vi "S2C_Access_MenuAct.vi"(8 "Error In":errorcluster, 11 "Coords":cluster{"Row":dbl, "Column":dbl}) -> (0 "Error Out":errorcluster, 2 "MenuItems":string[](array[string]), 3 "Discard?":bool)   [LabVIEW 2015]
uses:
  S2C_Access_Globals.vi
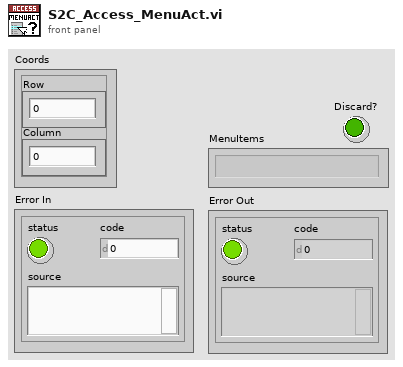
[diagram p1: front panel]
types:
  T1 = typedef "LVRowAndColumnTypeDef.ctl" = cluster{"Row":i32, "Column":i32}
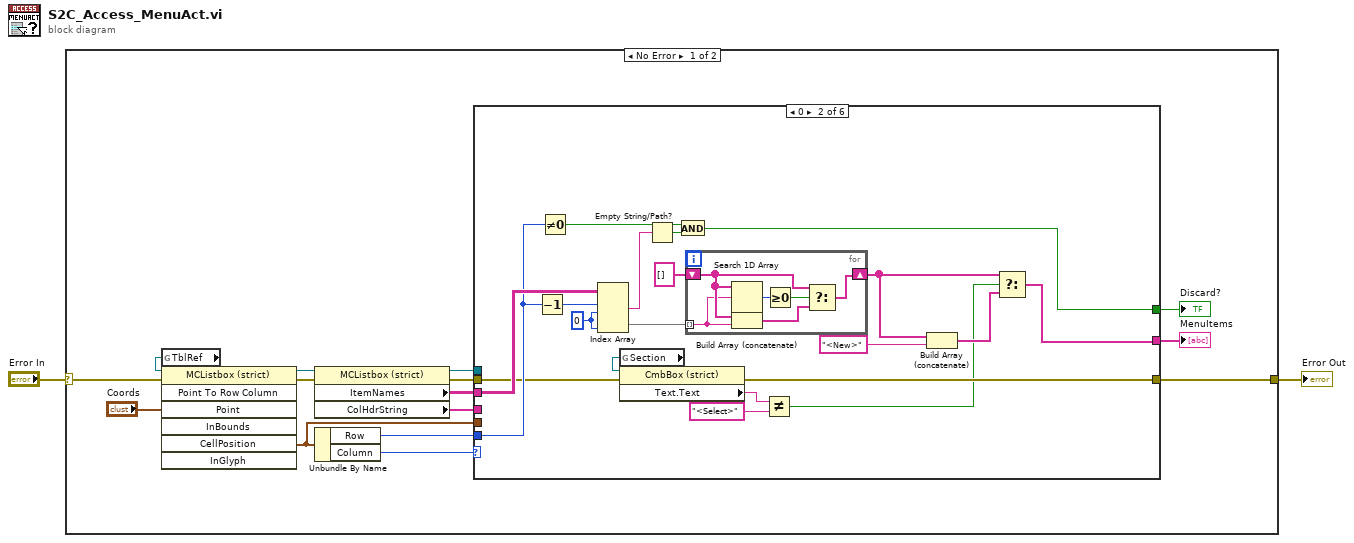
[diagram p0: block diagram]
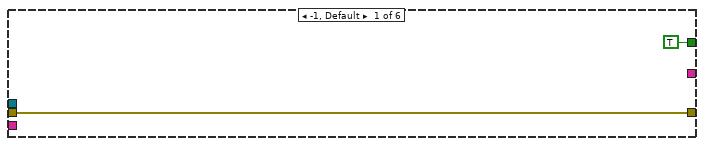
[diagram p2: hidden frame]
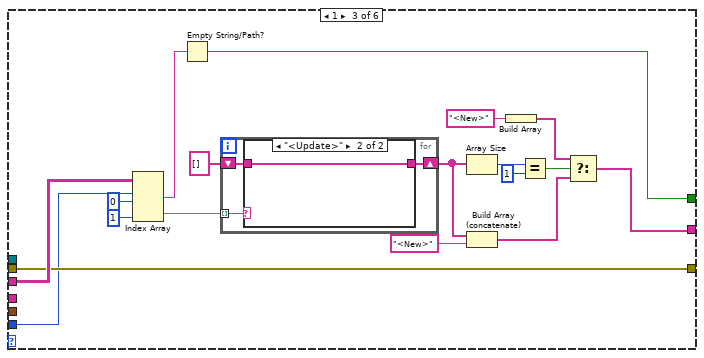
[diagram p3: hidden frame]
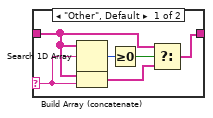
[diagram p4: hidden frame]
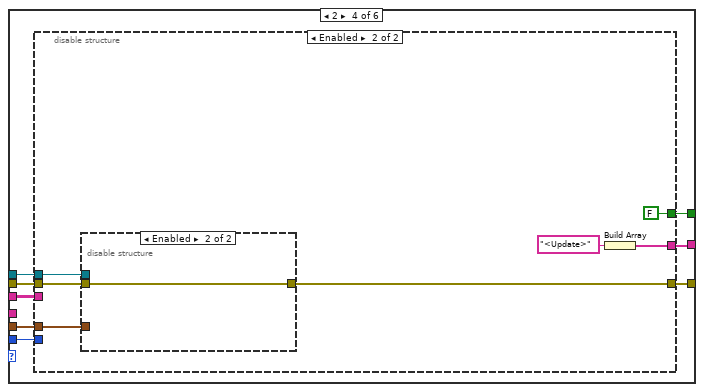
[diagram p5: hidden frame]
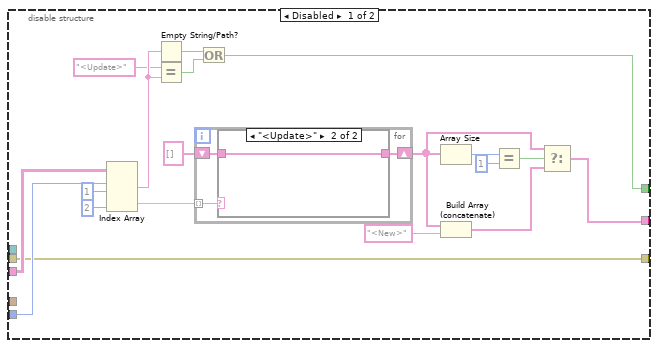
[diagram p6: hidden frame]
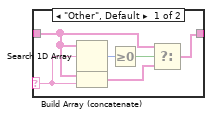
[diagram p7: hidden frame]
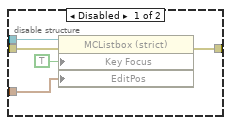
[diagram p8: hidden frame]
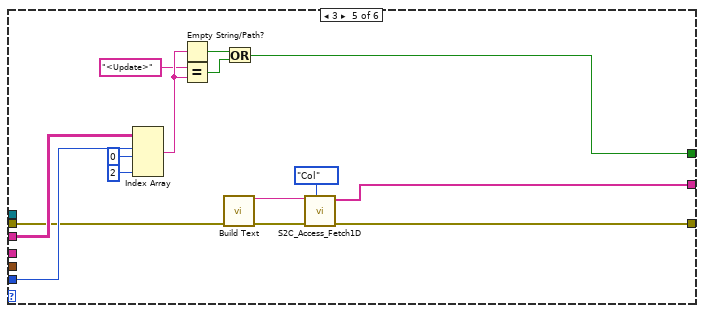
[diagram p9: hidden frame]
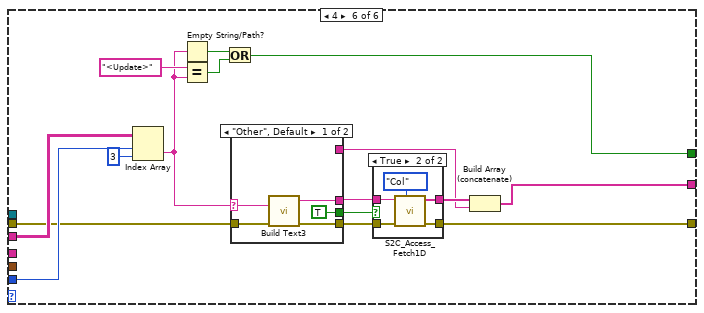
[diagram p10: hidden frame]
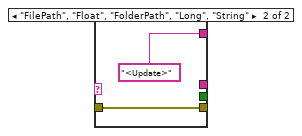
[diagram p12: hidden frame]
diagram:
  n1 = case shown="No Error" "Error In" {
    selector: "Error In" -> [w7 w168]
    tunnel: [w6 w168] -> w1
    frame No Error {
      n2 = global read "S2C_Access_Globals.vi" "TblRef"() -> (w17:refnum<vi>)
      n3 = invoke class="MCListbox (strict)" method="Point To Row Column"(reference=w17, error in=w7, "Point"="Coords") -> (reference out=w14:refnum<vi>, error out=w15:errorcluster, "CellPosition"=w3:T1)  [unwired: 4 in, 4 out]
      n4 = property class="MCListbox (strict)"(reference=w14, error in=w15) -> (reference out=w4:refnum<vi>, error out=w13:errorcluster, "ItemNames"=w10:string[][], "ColHdrString"=w9:string[])
      n5 = Unbundle By Name(w3) -> ("Row"=w11:i32, "Column"=w12:i32)
      n6 = case shown="0" w12 {
        tunnel: w13 -> [w19 w31 w59 w77 w129 w147]
        tunnel: w11 -> [_ w34 w56 w80 w135 w152]
        tunnel: w10 -> [_ w39 w63 w81 w138 w154]
        tunnel: w9 -> [_ _ _ _ _ _]
        tunnel: [TRUE w30 w55 w79 w130 w148] -> w8
        tunnel: [w19 w24 w59 w76 w125 w141] -> w6
        tunnel: [_ w25 w48 w78 w126 w140] -> w5
        tunnel: w4 -> [_ _ _ w75 _ _]
        tunnel: w3 -> [_ _ _ w74 _ _]
        frame -1, Default {
        }
        frame 0 {
          w29 = 0 ("disabled index (col)")
          n7 = Decrement(x=w34) -> (x-1=w38:i32)
          n8 = Not Equal To 0?(x=w34) -> (x != 0?=w35:bool)
          n9 = Index Array(array=w39, index (row) #1=w38, index (col) #1=w29, index (col) #2=w29) -> (element #1=w37:string, element #2=w33:string[])  [unwired: 1 in]
          n10 = global read "S2C_Access_Globals.vi" "Section"() -> (w23:refnum<vi>)
          n11 = property class="CmbBox (strict)"(reference=w23, error in=w31) -> (error out=w24:errorcluster, "Text.Text"=w22:string)  [unwired: 1 out]
          n12 = Empty String/Path?(string/path=w37) -> (empty?=w36:bool)
          n13 = And(x=w35, y=w36) -> (x .and. y?=w30:bool)
          n14 = for {
            tunnel: w33 -> [w40] mode=indexing
            shift-right: [w43] -> w28
            shift-left: string[] [] ("Array - String") -> [w42]
            n15 = Search 1D Array(1D array=w42, element=w40) -> (index of element=w45:i32)  [unwired: 1 in]
            n16 = Build Array (concatenate)(w42, w40) -> (w41:string[])
            n17 = Greater Or Equal To 0?(x=w45) -> (x >= 0?=w44:bool)
            n18 = Select(t=w42, s=w44, f=w41) -> (s? t:f=w43:string[])
          }
          n19 = Not Equal?(x=w22, y="<Select>") -> (x != y?=w20:bool)
          n20 = Build Array (concatenate)(w28, "<New>") -> (w26:string[])
          n21 = Select(t=w28, s=w20, f=w26) -> (s? t:f=w25:string[])
        }
        frame 1 {
          n22 = Index Array(array=w63, index (row) #1=w56, index (col) #1=0 ("disabled index (col)"), index (col) #2=1 ("index (col)")) -> (element #1=w62:string, element #2=w61:string[])  [unwired: 1 in]
          n23 = Empty String/Path?(string/path=w62) -> (empty?=w55:bool)
          n24 = for {
            tunnel: w61 -> [w64] mode=indexing
            shift-right: [w66] -> w50
            shift-left: string[] [] ("Array - String") -> [w65]
            n25 = case shown="\"<Update>\"" w64 {
              selector: w64 -> [w67 _]
              tunnel: [w70 w73] -> w66
              tunnel: w65 -> [w69 w73]
              frame "Other", Default {
                n26 = Search 1D Array(1D array=w69, element=w67) -> (index of element=w72:i32)  [unwired: 1 in]
                n27 = Build Array (concatenate)(w69, w67) -> (w68:string[])
                n28 = Greater Or Equal To 0?(x=w72) -> (x >= 0?=w71:bool)
                n29 = Select(t=w69, s=w71, f=w68) -> (s? t:f=w70:string[])
              }
              frame "<Update>" {
              }
            }
          }
          n30 = Array Size(array=w50) -> (size(s)=w53:i32)
          n31 = Build Array (concatenate)(w50, "<New>") -> (w49:string[])
          n32 = Build Array("<New>") -> (w46:string[])
          n33 = Equal?(x=w53, y=1) -> (x = y?=w51:bool)
          n34 = Select(t=w46, s=w51, f=w49) -> (s? t:f=w48:string[])
        }
        frame 2 {
          n35 = disable-structure shown="Enabled" {
            disable-tunnel: w81 -> [w100 _]
            disable-tunnel: w80 -> [w97 _]
            disable-tunnel: [w92 FALSE] -> w79
            disable-tunnel: [w83 w111] -> w78
            disable-tunnel: w77 -> [w82 w117]
            disable-tunnel: [w82 w114] -> w76
            disable-tunnel: w75 -> [_ w116]
            disable-tunnel: w74 -> [_ w115]
            frame Disabled {
              n36 = Index Array(array=w100, index (row) #1=w97, index (col) #1=1 ("disabled index (col)"), index (col) #2=2 ("index (col)")) -> (element #1=w96:string, element #2=w84:string[])  [unwired: 1 in]
              n37 = Empty String/Path?(string/path=w96) -> (empty?=w93:bool)
              n38 = Equal?(x="<Update>", y=w96) -> (x = y?=w94:bool)
              n39 = for {
                tunnel: w84 -> [w101] mode=indexing
                shift-right: [w103] -> w86
                shift-left: string[] [] ("Array - String") -> [w102]
                n40 = case shown="\"<Update>\"" w101 {
                  selector: w101 -> [w104 _]
                  tunnel: [w107 w110] -> w103
                  tunnel: w102 -> [w106 w110]
                  frame "Other", Default {
                    n41 = Search 1D Array(1D array=w106, element=w104) -> (index of element=w109:i32)  [unwired: 1 in]
                    n42 = Build Array (concatenate)(w106, w104) -> (w105:string[])
                    n43 = Greater Or Equal To 0?(x=w109) -> (x >= 0?=w108:bool)
                    n44 = Select(t=w106, s=w108, f=w105) -> (s? t:f=w107:string[])
                  }
                  frame "<Update>" {
                  }
                }
              }
              n45 = Or(x=w93, y=w94) -> (x .or. y?=w92:bool)
              n46 = Array Size(array=w86) -> (size(s)=w89:i32)
              n47 = Build Array (concatenate)(w86, "<New>") -> (w85:string[])
              n48 = Equal?(x=w89, y=1) -> (x = y?=w87:bool)
              n49 = Select(t=w86, s=w87, f=w85) -> (s? t:f=w83:string[])
            }
            frame Enabled {
              n50 = disable-structure shown="Enabled" {
                disable-tunnel: w117 -> [w122 w123]
                disable-tunnel: w116 -> [w121 _]
                disable-tunnel: w115 -> [w119 _]
                disable-tunnel: [w118 w123] -> w114
                frame Disabled {
                  n51 = property class="MCListbox (strict)"(reference=w121, error in=w122, "Key Focus"=TRUE, "EditPos"=w119) -> (error out=w118:errorcluster)  [unwired: 1 out]
                }
                frame Enabled {
                }
              }
              n52 = Build Array("<Update>") -> (w111:string[])
            }
          }
        }
        frame 3 {
          n53 = Index Array(array=w138, index (row) #1=w135, index (col) #1=0 ("disabled index (col)"), index (col) #2=2 ("index (col)")) -> (element #1=w134:string)  [unwired: 1 in, 1 out]
          n54 = Empty String/Path?(string/path=w134) -> (empty?=w131:bool)
          n55 = Equal?(x="<Update>", y=w134) -> (x = y?=w132:bool)
          n56 = call "Build Text"("error in (no error)"=w129) -> ("Result"=w127:string, "error out"=w128:errorcluster)  [unwired: 13 in]
          n57 = Or(x=w131, y=w132) -> (x .or. y?=w130:bool)
          n58 = call "S2C_Access_Fetch1D.vi"("Selection"=enum16{"Row", "Col"}."Col", "Error In"=w128, "Query"=w127) -> ("Error Out"=w125:errorcluster, "Data"=w126:string[])  [unwired: 7 in]
        }
        frame 4 {
          n59 = Index Array(array=w154, index (row)=w152, index (col)=3 ("disabled index (col)")) -> (element=w139:string)
          n60 = Empty String/Path?(string/path=w139) -> (empty?=w149:bool)
          n61 = Equal?(x="<Update>", y=w139) -> (x = y?=w150:bool)
          n62 = Or(x=w149, y=w150) -> (x .or. y?=w148:bool)
          n63 = case shown="\"Other\", Default" w139 {
            selector: w139 -> [w162 _]
            tunnel: w147 -> [w165 w167]
            tunnel: [w164 w167] -> w146
            tunnel: [w163 _] -> w145
            tunnel: [_ "<Update>"] -> w142
            tunnel: [TRUE _] -> w144
            frame "Other", Default {
              n64 = call "Build Text3"("Section"=w162, "error in (no error)"=w165) -> ("Result"=w163:string, "error out"=w164:errorcluster)  [unwired: 12 in]
            }
            frame "FilePath", "Float", "FolderPath", "Long", "String" {
            }
          }
          n65 = case shown="True" w144 {
            tunnel: w146 -> [w155 w160]
            tunnel: [w155 w159] -> w141
            tunnel: [_ w158] -> w143
            tunnel: w145 -> [_ w157]
            frame False {
            }
            frame True {
              n66 = call "S2C_Access_Fetch1D.vi"("Selection"=enum16{"Row", "Col"}."Col", "Error In"=w160, "Query"=w157) -> ("Error Out"=w159:errorcluster, "Data"=w158:string[])  [unwired: 7 in]
            }
          }
          n67 = Build Array (concatenate)(w143, w142) -> (w140:string[])
        }
      }
      "MenuItems" <- w5
      "Discard?" <- w8
    }
    frame Error {
    }
  }
  "Error Out" <- w1
